vi "oa_Config Scale and Unit for Cascade Plot.vi"(0 "cascade plot ref":refnum<vi>, 1 "plot type":T1(ring), 5 "scales":T3 {"Y scale"."multiplier" format="%.2f"; "Y scale"."offset" format="%.2f"; "X scale"."multiplier" format="%.2f"; "X scale"."offset" format="%.2f"}, 7 "unit labels":T2, 9 "spectral map":dbl[][](array[numeric]) format="%.2f", 11 "error in (no error)":errorcluster, 12 "dB on":bool=TRUE) -> (4 "cascade plot ref out":refnum<vi>, 6 "X scale":cluster{"offset":dbl, "multiplier":dbl} {"multiplier" format="%.2f"; "offset" format="%.2f"}, 8 "Y scale":cluster{"offset":dbl, "multiplier":dbl} {"multiplier" format="%.2f"; "offset" format="%.2f"}, 10 "spectral map out":dbl[][](array[numeric]) format="%.2f", 15 "error out":errorcluster)   [LabVIEW 2017]
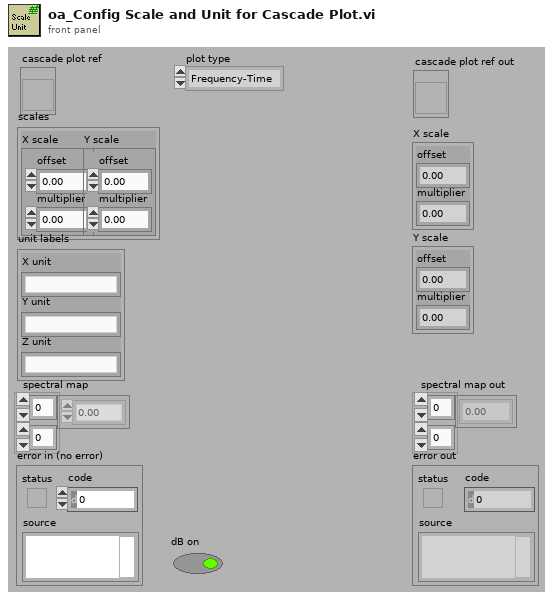
[diagram p1: front panel]
types:
  T1 = enum16{"Frequency-Time", "Time-Frequency", "Order-Time", "Time-Order", "Frequency-RPM", "RPM-Frequency", "Order-RPM", "RPM-Order"}
  T2 = cluster{"X unit":string, "Y unit":string, "Z unit":string}
  T3 = cluster{"X scale":cluster{"offset":dbl, "multiplier":dbl}, "Y scale":cluster{"offset":dbl, "multiplier":dbl}}
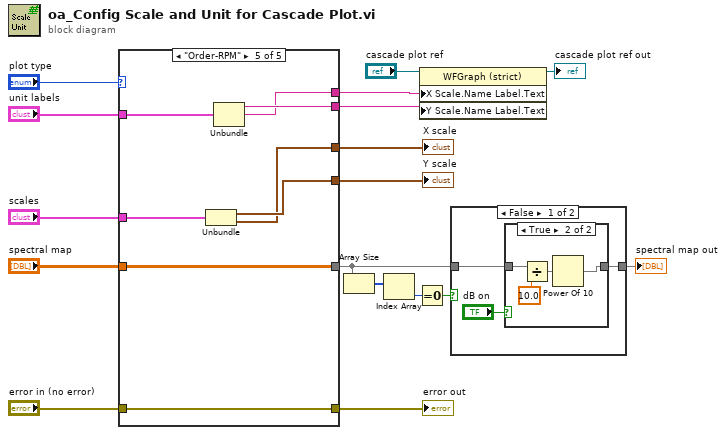
[diagram p0: block diagram]
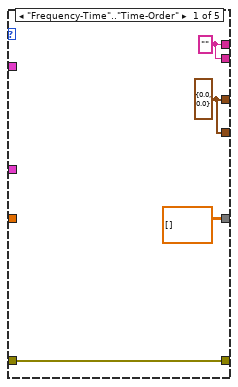
[diagram p4: hidden frame]
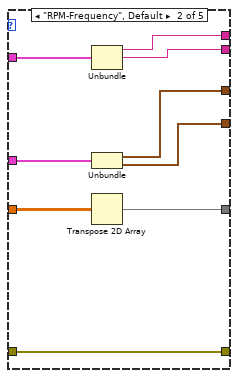
[diagram p5: hidden frame]
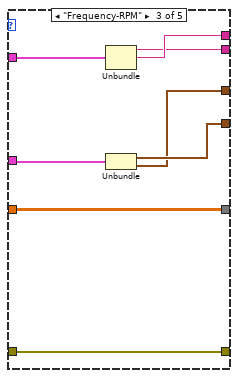
[diagram p6: hidden frame]
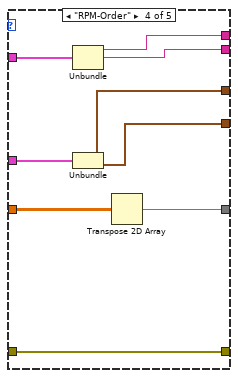
[diagram p7: hidden frame]
diagram:
  n1 = case shown="\"Order-RPM\"" "plot type" {
    tunnel: "scales" -> [_ w30 w38 w47 w55]
    tunnel: [w20 w28 w37 w46 w54] -> w15
    tunnel: [w20 w29 w36 w45 w53] -> w14
    tunnel: "unit labels" -> [_ w27 w35 w44 w52]
    tunnel: [w21 w26 w34 w43 w50] -> w12
    tunnel: [w21 w25 w33 w42 w51] -> w11
    tunnel: "spectral map" -> [_ w24 w32 w41 w49]
    tunnel: [dbl[][] [] ("spectral map") w23 w32 w40 w49] -> w2
    tunnel: "error in (no error)" -> [w18 w22 w31 w39 w48]
    tunnel: [w18 w22 w31 w39 w48] -> w6
    frame "Frequency-Time".."Time-Order" {
      w21 = ""
      w20 = cluster{"offset":dbl, "multiplier":dbl} {"offset"=0.0, "multiplier"=0.0}
    }
    frame "RPM-Frequency", Default {
      n2 = Unbundle(w27) -> ("X unit"=w26:string, "Y unit"=w25:string)  [unwired: 1 out]
      n3 = Unbundle(w30) -> ("X scale"=w29:cluster{"offset":dbl, "multiplier":dbl}, "Y scale"=w28:cluster{"offset":dbl, "multiplier":dbl})
      n4 = Transpose 2D Array(2D array=w24) -> (transposed array=w23:dbl[][])
    }
    frame "Frequency-RPM" {
      n5 = Unbundle(w35) -> ("X unit"=w33:string, "Y unit"=w34:string)  [unwired: 1 out]
      n6 = Unbundle(w38) -> ("X scale"=w37:cluster{"offset":dbl, "multiplier":dbl}, "Y scale"=w36:cluster{"offset":dbl, "multiplier":dbl})
    }
    frame "RPM-Order" {
      n7 = Unbundle(w44) -> ("X unit"=w43:string, "Y unit"=w42:string)  [unwired: 1 out]
      n8 = Unbundle(w47) -> ("X scale"=w45:cluster{"offset":dbl, "multiplier":dbl}, "Y scale"=w46:cluster{"offset":dbl, "multiplier":dbl})
      n9 = Transpose 2D Array(2D array=w41) -> (transposed array=w40:dbl[][])
    }
    frame "Order-RPM" {
      n10 = Unbundle(w55) -> ("X scale"=w54:cluster{"offset":dbl, "multiplier":dbl}, "Y scale"=w53:cluster{"offset":dbl, "multiplier":dbl})
      n11 = Unbundle(w52) -> ("X unit"=w51:string, "Y unit"=w50:string)  [unwired: 1 out]
    }
  }
  "X scale" <- w14
  "Y scale" <- w15
  "error out" <- w6
  n12 = Array Size(array=w2) -> (size(s)=w5:i32[])
  n13 = Index Array(array=w5) -> (element=w4:i32)  [unwired: 1 in]
  n14 = Equal To 0?(x=w4) -> (x = 0?=w3:bool)
  n15 = property class="WFGraph (strict)"(reference="cascade plot ref", "X Scale.Name Label.Text"=w12, "Y Scale.Name Label.Text"=w11) -> (reference out=→"cascade plot ref out":refnum<vi>)  [unwired: 1 in, 1 out]
  n16 = case shown="False" w3 {
    tunnel: w2 -> [w58 w64]
    tunnel: [w56 w64] -> w1
    frame False {
      n17 = case shown="True" "dB on" {
        tunnel: w58 -> [w59 w63]
        tunnel: [w59 w60] -> w56
        frame False {
        }
        frame True {
          n18 = Divide(x=w63, y=10.0) -> (x/y=w61:dbl[][])
          n19 = Power Of 10(x=w61) -> (10^x=w60:dbl[][])
        }
      }
    }
    frame True {
    }
  }
  "spectral map out" <- w1
